vi "GraphPanUpdate.vi"(8 "error in (no error)":errorcluster caption="entrée d'erreur (pas d'erreur)", 9 "GraphInd":i32[](array[numeric]), 10 "DeferUpdate":bool, 11 "Interface en entrée":refnum<class "Interface.lvclass"> caption="DNL_LabVIEW Object in") -> (0 "error out":errorcluster caption="sortie d'erreur", 3 "Interface en sortie":refnum<class "Interface.lvclass"> caption="DNL_LabVIEW Object out")   [LabVIEW 2019, in "Interface.lvclass"]
uses:
  Interface.lvclass
  Interface.lvclass/Interface.ctl
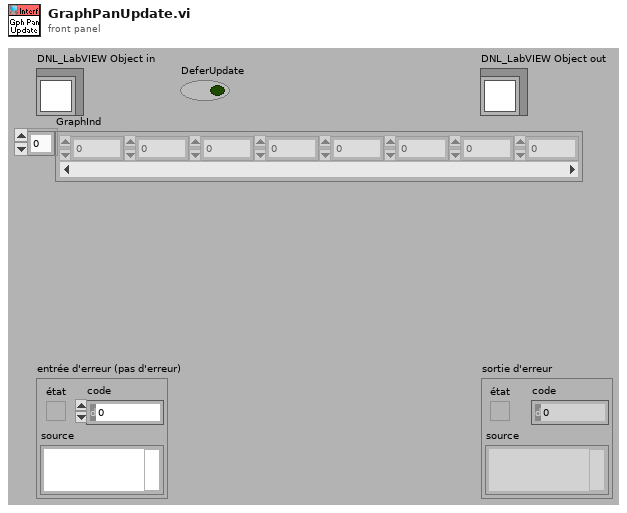
[diagram p1: front panel]
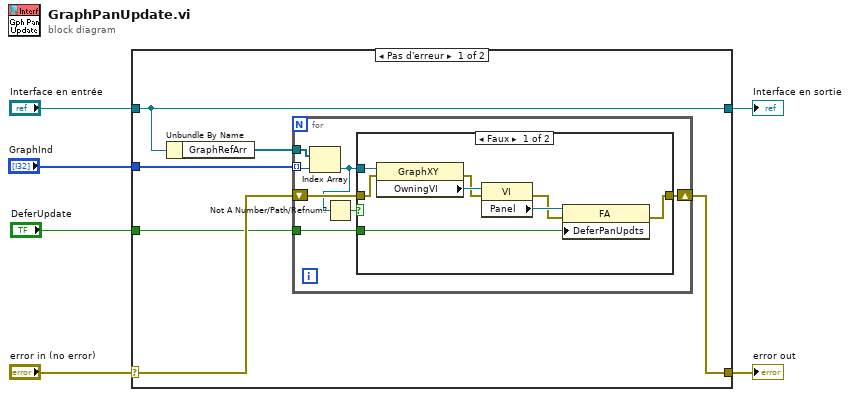
[diagram p0: block diagram]
diagram:
  n1 = case shown="Pas d'erreur" "error in (no error)" {
    selector: "error in (no error)" -> [w11 w30]
    tunnel: [w9 w30] -> w5
    tunnel: [w12 w29] -> w3
    tunnel: "Interface en entrée" -> [w12 w29]
    tunnel: "DeferUpdate" -> [w8 _]
    tunnel: "GraphInd" -> [w7 _]
    frame No Error {
      n2 = Unbundle By Name(w12) -> ("GraphRefArr"=w10:refnum<vi>[])
      n3 = for {
        shift-right: [w18] -> w9
        shift-left: w11 -> [w19]
        tunnel: w10 -> [w17]
        tunnel: w7 -> [w16] mode=indexing
        tunnel: w8 -> [w15]
        n4 = Index Array(array=w17, index=w16) -> (element=w13:refnum<vi>)
        n5 = Not A Number/Path/Refnum?(number/path/refnum=w13) -> (NaN/Path/Refnum?=w14:bool)
        n6 = case shown="Faux" w14 {
          tunnel: w19 -> [w26 w28]
          tunnel: [w22 w28] -> w18
          tunnel: w13 -> [w21 _]
          tunnel: w15 -> [w20 _]
          frame False {
            n7 = property class="GraphXY"(reference=w21, error in=w26) -> (error out=w25:errorcluster, "OwningVI"=w27:refnum<vi>)  [unwired: 1 out]
            n8 = property class="VI"(reference=w27, error in=w25) -> (error out=w23:errorcluster, "Panel"=w24:refnum<vi>)  [unwired: 1 out]
            n9 = property class="FA"(reference=w24, error in=w23, "DeferPanUpdts"=w20) -> (error out=w22:errorcluster)  [unwired: 1 out]
          }
          frame True {
          }
        }
      }
    }
    frame Error {
    }
  }
  "error out" <- w5
  "Interface en sortie" <- w3
